vi "Process Data.vi"(8 "error in":errorcluster, 11 "Broker in":refnum<class "Broker.lvclass">) -> (0 "error out":errorcluster, 3 "Broker out":refnum<class "Broker.lvclass">)   [LabVIEW 2014, in "Broker.lvclass"]
uses:
  Broker.lvclass
  Topic_class/Topic.lvclass
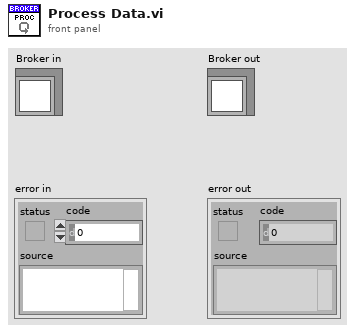
[diagram p1: front panel]
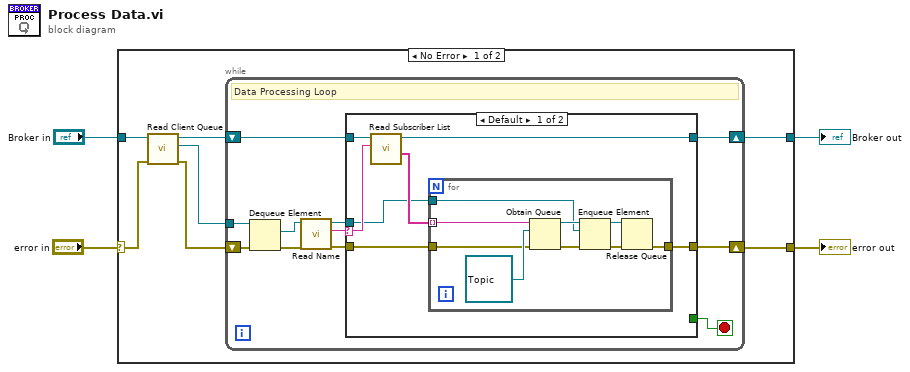
[diagram p0: block diagram]
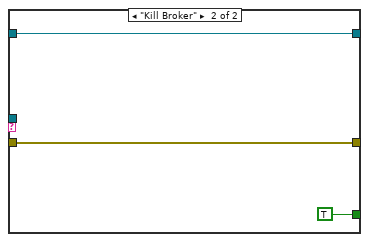
[diagram p2: hidden frame]
diagram:
  n1 = case shown="No Error" "error in" {
    selector: "error in" -> [w5 w43]
    tunnel: [w6 w43] -> w1
    tunnel: [w8 w42] -> w3
    tunnel: "Broker in" -> [w11 w42]
    frame No Error {
      n2 = call-dynamic "Read Client Queue.vi"("error in"=w5, "Client in"=w11) -> ("error out"=w7:errorcluster, "Client Queue"=w10:refnum<queue>, "Client out"=w9:refnum<class "Broker.lvclass">)  [unwired: 7 in]
      n3 = while {
        tunnel: w10 -> [w22]
        shift-right: [w14] -> w8
        shift-left: w9 -> [w15]
        shift-right: [w12] -> w6
        shift-left: w7 -> [w13]
        stop <- w16 stop-if-true
        # "Data Processing Loop"
        n4 = Dequeue Element(queue=w22, error in (no error)=w13) -> (element=w20:refnum<class "Topic.lvclass">, error out=w21:errorcluster)  [unwired: 1 in, 2 out]
        n5 = call-dynamic "Read Name.vi"("error in"=w21, "Topic in"=w20) -> ("error out"=w18:errorcluster, "Name"=w19:string, "Topic out"=w17:refnum<class "Topic.lvclass">)  [unwired: 7 in]
        n6 = case shown="Default" w19 {
          selector: w19 -> [w27 _]
          tunnel: [_ TRUE] -> w16
          tunnel: w18 -> [w26 w40]
          tunnel: [w25 w40] -> w12
          tunnel: w17 -> [w23 _]
          tunnel: w15 -> [w29 w39]
          tunnel: [w28 w39] -> w14
          frame Default {
            n7 = call-dynamic "Read Subscriber List.vi"("Topic Name"=w27, "Broker in"=w29) -> ("Subscriber List"=w24:string[], "Broker out"=w28:refnum<class "Broker.lvclass">)  [unwired: 6 in, 2 out]
            n8 = for {
              tunnel: w26 -> [w35]
              tunnel: [w32] -> w25
              tunnel: w24 -> [w31] mode=indexing
              tunnel: w23 -> [w30]
              n9 = Obtain Queue(name (unnamed)=w31, element data type=refnum<class "Topic.lvclass"> refnum ("Topic.lvclass"), error in (no error)=w35) -> (queue out=w37:refnum<queue>, error out=w34:errorcluster)  [unwired: 2 in, 1 out]
              n10 = Enqueue Element(queue=w37, element=w30, error in (no error)=w34) -> (queue out=w36:refnum<queue>, error out=w33:errorcluster)  [unwired: 1 in, 1 out]
              n11 = Release Queue(queue=w36, error in (no error)=w33) -> (error out=w32:errorcluster)  [unwired: 1 in, 2 out]
            }
          }
          frame "Kill Broker" {
          }
        }
      }
    }
    frame Error {
    }
  }
  "error out" <- w1
  "Broker out" <- w3
